vi "CreateDAQDict.vi"(8 "error in (no error)":errorcluster, 10 "IO Tasks[]":T1[](array[typedef])=[{"IO Type"=enum."DI", "TaskID"="DI_TaskID_C1", "IONames"=["DI1_00_Main Photohelic Pressure Low", "DI1_01_Main Photohelic Pressure High", "DI1_02_Main E-Stop Circuit OK", "DI1_03_EMO Circuit OK", "DI1_04_Nitrogen Top Valve Open", "DI1_05_Nitrogen Bottom Valve Open", "DI1_06_Nitrogen Pressure OK", "DI1_07_CDA Pressure OK", "DI1_08_Vacuum OK", "DI1_09_Aligner Home", "DI1_10_Aligner Reticle Present", "DI1_11_Main Door Interlock Solenoid Closed", "DI1_12_Main Door Closed", "DI1_13_Main Robot $ALARM_STOP", "DI1_14_Main Robot $IN_HOME", "DI1_15_Main Robot $PERI_RDY", "DI1_16_Main Robot $TCP_OPEN", "DI1_17_Main End Eff Open", "DI1_18_Main End Eff Closed", "DI1_19_Main Reticle Presence sensor-Arm-Right", "DI1_20_Spare_1", "DI1_21_Main Reticle Presence sensor-Arm-Left", "DI1_22_EXP1 XFR Reticle Present", "DI1_23_EXP2 XFR Reticle Present", "DI1_24_Main Robot $EXT (External Mode ON)", "DI1_25_Main Robot $PRO_ACT (Program Active)", "DI1_26_Main Robot $PRO_MOVE (Motion Active)", "DI1_27_Main Robot Spare1", "DI1_28_Main Robot Spare2", "DI1_29_Main Robot Spare3", "DI1_30_Spare_2", "DI1_31_Spare_3", "DI2_00_ASML_RSP LP 1 Pod Presence", "DI2_01_Spare_4", "DI2_02_ASML_RSP LP 2 Pod Presence", "DI2_03_Spare_5", "DI2_04_ASML_RSP LP 3 Pod Presence", "DI2_05_Spare_6", "DI2_06_Spare_7", "DI2_07_Manual Loadport 1 Pod Present", "DI2_08_Manual Loadport 1 Pod Capture", "DI2_09_Manual Loadport 1 Arm in Open Position", "DI2_10_Manual Loadport 1 Arm in Closed Position", "DI2_11_Manual Loadport 1 Lid Capture", "DI2_12_Manual Loadport 1 Door Closed", "DI2_13_Manual Loadport 1 Reticle Present", "DI2_14_Manual Loadport 1 Lid Present on Arm", "DI2_15_MLP Spare Input", "DI2_16_Pod Buffer Inbound Pod Present", "DI2_17_Pod Buffer Outbound Pod Present", "DI2_18_Pod Buffer Door Closed", "DI2_19_Pod Buffer Light Curtain OK", "DI2_20_Pod Buffer Light Curtain Misc Input", "DI2_21_Pod Buffer Gripper Pod Present", "DI2_22_Pod Buffer Gripper open", "DI2_23_Pod Buffer Gripper closed", "DI2_24_FFU Pressure sensor 1", "DI2_25_FFU Pressure sensor 2", "DI2_26_FFU Pressure sensor 3", "DI2_27_FFU Pressure sensor 4", "DI2_28_FFU Pressure sensor 5", "DI2_29_FFU Pressure sensor 6", "DI2_30_FFU Pressure sensor 7", "DI2_31_FFU Pressure sensor 8"], "ChPath"=["C1M1_9425_DI1/Port0/Line0", "C1M1_9425_DI1/Port0/Line1", "C1M1_9425_DI1/Port0/Line2", "C1M1_9425_DI1/Port0/Line3", "C1M1_9425_DI1/Port0/Line4", "C1M1_9425_DI1/Port0/Line5", "C1M1_9425_DI1/Port0/Line6", "C1M1_9425_DI1/Port0/Line7", "C1M1_9425_DI1/Port0/Line8", "C1M1_9425_DI1/Port0/Line9", "C1M1_9425_DI1/Port0/Line10", "C1M1_9425_DI1/Port0/Line11", "C1M1_9425_DI1/Port0/Line12", "C1M1_9425_DI1/Port0/Line13", "C1M1_9425_DI1/Port0/Line14", "C1M1_9425_DI1/Port0/Line15", "C1M1_9425_DI1/Port0/Line16", "C1M1_9425_DI1/Port0/Line17", "C1M1_9425_DI1/Port0/Line18", "C1M1_9425_DI1/Port0/Line19", "C1M1_9425_DI1/Port0/Line20", "C1M1_9425_DI1/Port0/Line21", "C1M1_9425_DI1/Port0/Line22", "C1M1_9425_DI1/Port0/Line23", "C1M1_9425_DI1/Port0/Line24", "C1M1_9425_DI1/Port0/Line25", "C1M1_9425_DI1/Port0/Line26", "C1M1_9425_DI1/Port0/Line27", "C1M1_9425_DI1/Port0/Line28", "C1M1_9425_DI1/Port0/Line29", "C1M1_9425_DI1/Port0/Line30", "C1M1_9425_DI1/Port0/Line31", "C1M2_9425_DI2/Port0/Line0", "C1M2_9425_DI2/Port0/Line1", "C1M2_9425_DI2/Port0/Line2", "C1M2_9425_DI2/Port0/Line3", "C1M2_9425_DI2/Port0/Line4", "C1M2_9425_DI2/Port0/Line5", "C1M2_9425_DI2/Port0/Line6", "C1M2_9425_DI2/Port0/Line7", "C1M2_9425_DI2/Port0/Line8", "C1M2_9425_DI2/Port0/Line9", "C1M2_9425_DI2/Port0/Line10", "C1M2_9425_DI2/Port0/Line11", "C1M2_9425_DI2/Port0/Line12", "C1M2_9425_DI2/Port0/Line13", "C1M2_9425_DI2/Port0/Line14", "C1M2_9425_DI2/Port0/Line15", "C1M2_9425_DI2/Port0/Line16", "C1M2_9425_DI2/Port0/Line17", "C1M2_9425_DI2/Port0/Line18", "C1M2_9425_DI2/Port0/Line19", "C1M2_9425_DI2/Port0/Line20", "C1M2_9425_DI2/Port0/Line21", "C1M2_9425_DI2/Port0/Line22", "C1M2_9425_DI2/Port0/Line23", "C1M2_9425_DI2/Port0/Line24", "C1M2_9425_DI2/Port0/Line25", "C1M2_9425_DI2/Port0/Line26", "C1M2_9425_DI2/Port0/Line27", "C1M2_9425_DI2/Port0/Line28", "C1M2_9425_DI2/Port0/Line29", "C1M2_9425_DI2/Port0/Line30", "C1M2_9425_DI2/Port0/Line31"], "Task Ref"=""}, {"IO Type"=enum."DI", "TaskID"="DI_TaskID_C2A", "IONames"=["DI3_00_Exp1 Photohelic Pressure Low", "DI3_01_Main Photohelic Pressure High", "DI3_02_Main E-Stop Circuit OK", "DI3_03_Spare_1", "DI3_04_Exp1 Door Interlock Solenoid Closed", "DI3_05_Exp1 Door Closed", "DI3_06_Spare_2", "DI3_07_Spare_3", "DI3_08_Spare_4", "DI3_09_Spare_5", "DI3_10_Exp1 End Eff Open", "DI3_11_Exp1 End Eff Closed", "DI3_12_Exp1 Reticle Presence sensor-Arm-Right", "DI3_13_Exp1 Robot $ALARM_STOP", "DI3_14_Exp1 Robot $IN_HOME", "DI3_15_Exp1 Robot $PERI_RDY", "DI3_16_Exp1 Robot $TCP_OPEN", "DI3_17_Exp1 Reticle Presence sensor-Arm-Left", "DI3_18_Exp1 FFU Pressure sensor 1", "DI3_19_Exp1 FFU Pressure sensor 2", "DI3_20_Exp1 FFU Pressure sensor 3", "DI3_21_Exp1 FFU Pressure sensor 4", "DI3_22_Exp1 FFU Pressure sensor 5", "DI3_23_Exp1 FFU Pressure sensor 6", "DI3_24_Exp1 Robot $EXT (External Mode ON)", "DI3_25_Exp1 Robot $PRO_ACT (Program Active)", "DI3_26_Exp1 Robot $PRO_MOVE (Motion Active)", "DI3_27_Exp1 FFU Pressure sensor 7", "DI3_28_Exp1 FFU Pressure sensor 8", "DI3_29_Exp1 output Spare 1", "DI3_30_Exp1 output Spare 2", "DI3_31_Exp1 output Spare 3"], "ChPath"=["C2AM1_9425_DI3/Port0/Line0", "C2AM1_9425_DI3/Port0/Line1", "C2AM1_9425_DI3/Port0/Line2", "C2AM1_9425_DI3/Port0/Line3", "C2AM1_9425_DI3/Port0/Line4", "C2AM1_9425_DI3/Port0/Line5", "C2AM1_9425_DI3/Port0/Line6", "C2AM1_9425_DI3/Port0/Line7", "C2AM1_9425_DI3/Port0/Line8", "C2AM1_9425_DI3/Port0/Line9", "C2AM1_9425_DI3/Port0/Line10", "C2AM1_9425_DI3/Port0/Line11", "C2AM1_9425_DI3/Port0/Line12", "C2AM1_9425_DI3/Port0/Line13", "C2AM1_9425_DI3/Port0/Line14", "C2AM1_9425_DI3/Port0/Line15", "C2AM1_9425_DI3/Port0/Line16", "C2AM1_9425_DI3/Port0/Line17", "C2AM1_9425_DI3/Port0/Line18", "C2AM1_9425_DI3/Port0/Line19", "C2AM1_9425_DI3/Port0/Line20", "C2AM1_9425_DI3/Port0/Line21", "C2AM1_9425_DI3/Port0/Line22", "C2AM1_9425_DI3/Port0/Line23", "C2AM1_9425_DI3/Port0/Line24", "C2AM1_9425_DI3/Port0/Line25", "C2AM1_9425_DI3/Port0/Line26", "C2AM1_9425_DI3/Port0/Line27", "C2AM1_9425_DI3/Port0/Line28", "C2AM1_9425_DI3/Port0/Line29", "C2AM1_9425_DI3/Port0/Line30", "C2AM1_9425_DI3/Port0/Line31"], "Task Ref"=""}, {"IO Type"=enum."DO", "TaskID"="DO_TaskID_C1", "IONames"=["DO1_00_Vacuum Circuit Enable", "DO1_01_Nitrogen Flow Valve Open", "DO1_02_Nitrogen Top Blow Off", "DO1_03_Nitrogen Bottom Blow Off", "DO1_04_Nitrogen Blow Off Exhaust Fan ON", "DO1_05_Signal Red Light", "DO1_06_Signal Amber Light", "DO1_07_Signal Green Light", "DO1_08_Signal Blue Light", "DO1_09_Robot Input spare 1", "DO1_10_Signal Flashing", "DO1_11_Door Interlock Solenoid Close", "DO1_12_Main Robot $CONF_MESS (Clear Error-Alarm)", "DO1_13_Main Robot $DRIVES_ON", "DO1_14_Main Robot $MOVE_ENABLE", "DO1_15_Main Robot $EXT_START (Start-Resume Program)", "DO1_16_Main Robot $DRIVES_OFF", "DO1_17_Robot Input Spare 2", "DO1_18_Robot Input Spare 3", "DO1_19_Robot Input Spare 4", "DO1_20_Robot Input Spare 5", "DO1_21_Pod Buffer Horiz Enable", "DO1_22_Pod Buffer Vert Enable", "DO1_23_Barcode Reader Backlight ON", "DO1_24_Digital Camera Image Capture", "DO1_25_BLIS ON", "DO1_26_Spare_1", "DO1_27_Spare_2", "DO1_28_Spare_3", "DO1_29_Spare_4", "DO1_30_Spare_5", "DO1_31_Spare_6", "DO2_00_Spare_7", "DO2_01_Spare_8", "DO2_02_Spare_9", "DO2_03_MLP1 Door Lock", "DO2_04_MLP1 Pod Capture", "DO2_05_MLP1 Lid Capture", "DO2_06_MLP1 Arm to Open position", "DO2_07_MLP1 Arm to Close position", "DO2_08_MLP1 Power On Indicator", "DO2_09_MLP1 Error Indicator", "DO2_10_MLP1 In Process Indicator", "DO2_11_Spare_10", "DO2_12_Spare_11", "DO2_13_Spare_12", "DO2_14_Spare_13", "DO2_15_Spare_14", "DO2_16_Spare_15", "DO2_17_Spare", "DO2_18_Spare", "DO2_19_Spare", "DO2_20_Spare", "DO2_21_Spare", "DO2_22_Spare", "DO2_23_Spare", "DO2_24_Spare", "DO2_25_Spare", "DO2_26_Spare", "DO2_27_Spare", "DO2_28_Spare", "DO2_29_Spare", "DO2_30_Spare", "DO2_31_Spare"], "ChPath"=["C1M3_9476_DO1/Port0/Line0", "C1M3_9476_DO1/Port0/Line1", "C1M3_9476_DO1/Port0/Line2", "C1M3_9476_DO1/Port0/Line3", "C1M3_9476_DO1/Port0/Line4", "C1M3_9476_DO1/Port0/Line5", "C1M3_9476_DO1/Port0/Line6", "C1M3_9476_DO1/Port0/Line7", "C1M3_9476_DO1/Port0/Line8", "C1M3_9476_DO1/Port0/Line9", "C1M3_9476_DO1/Port0/Line10", "C1M3_9476_DO1/Port0/Line11", "C1M3_9476_DO1/Port0/Line12", "C1M3_9476_DO1/Port0/Line13", "C1M3_9476_DO1/Port0/Line14", "C1M3_9476_DO1/Port0/Line15", "C1M3_9476_DO1/Port0/Line16", "C1M3_9476_DO1/Port0/Line17", "C1M3_9476_DO1/Port0/Line18", "C1M3_9476_DO1/Port0/Line19", "C1M3_9476_DO1/Port0/Line20", "C1M3_9476_DO1/Port0/Line21", "C1M3_9476_DO1/Port0/Line22", "C1M3_9476_DO1/Port0/Line23", "C1M3_9476_DO1/Port0/Line24", "C1M3_9476_DO1/Port0/Line25", "C1M3_9476_DO1/Port0/Line26", "C1M3_9476_DO1/Port0/Line27", "C1M3_9476_DO1/Port0/Line28", "C1M3_9476_DO1/Port0/Line29", "C1M3_9476_DO1/Port0/Line30", "C1M3_9476_DO1/Port0/Line31", "C1M4_9476_DO2/Port0/Line0", "C1M4_9476_DO2/Port0/Line1", "C1M4_9476_DO2/Port0/Line2", "C1M4_9476_DO2/Port0/Line3", "C1M4_9476_DO2/Port0/Line4", "C1M4_9476_DO2/Port0/Line5", "C1M4_9476_DO2/Port0/Line6", "C1M4_9476_DO2/Port0/Line7", "C1M4_9476_DO2/Port0/Line8", "C1M4_9476_DO2/Port0/Line9", "C1M4_9476_DO2/Port0/Line10", "C1M4_9476_DO2/Port0/Line11", "C1M4_9476_DO2/Port0/Line12", "C1M4_9476_DO2/Port0/Line13", "C1M4_9476_DO2/Port0/Line14", "C1M4_9476_DO2/Port0/Line15", "C1M4_9476_DO2/Port0/Line16", "C1M4_9476_DO2/Port0/Line17", "C1M4_9476_DO2/Port0/Line18", "C1M4_9476_DO2/Port0/Line19", "C1M4_9476_DO2/Port0/Line20", "C1M4_9476_DO2/Port0/Line21", "C1M4_9476_DO2/Port0/Line22", "C1M4_9476_DO2/Port0/Line23", "C1M4_9476_DO2/Port0/Line24", "C1M4_9476_DO2/Port0/Line25", "C1M4_9476_DO2/Port0/Line26", "C1M4_9476_DO2/Port0/Line27", "C1M4_9476_DO2/Port0/Line28", "C1M4_9476_DO2/Port0/Line29", "C1M4_9476_DO2/Port0/Line30", "C1M4_9476_DO2/Port0/Line31"], "Task Ref"=""}, {"IO Type"=enum."DO", "TaskID"="DO_TaskID_C2B", "IONames"=["DO3_00_Exp1 Door Lock Solenoid Close", "DO3_01_Spare", "DO3_02_Spare", "DO3_03_Spare", "DO3_04_Spare", "DO3_05_Spare", "DO3_06_Exp1 Input Spare 1", "DO3_07_Exp1 Input Spare 2", "DO3_08_Exp1 Input Spare 3", "DO3_09_Exp1 Input Spare 4", "DO3_10_Exp1 Input Spare 5", "DO3_11_Spare", "DO3_12_Exp1 Robot $CONF_MESS (Clear Error-Alarm)", "DO3_13_Exp1 Robot $DRIVES_ON", "DO3_14_Exp1 Robot $MOVE_ENABLE", "DO3_15_Exp1 Robot $EXT_START (Start-Resume Program)", "DO3_16_Exp1 Robot $DRIVES_OFF", "DO3_17_Spare", "DO3_18_Spare", "DO3_19_Spare", "DO3_20_Spare", "DO3_21_Spare", "DO3_22_Spare", "DO3_23_Spare", "DO3_24_Spare", "DO3_25_Spare", "DO3_26_Spare", "DO3_27_Spare", "DO3_28_Spare", "DO3_29_Spare", "DO3_30_Spare", "DO3_31_Spare"], "ChPath"=["C2BM1_9476_DO3/Port0/Line0", "C2BM1_9476_DO3/Port0/Line1", "C2BM1_9476_DO3/Port0/Line2", "C2BM1_9476_DO3/Port0/Line3", "C2BM1_9476_DO3/Port0/Line4", "C2BM1_9476_DO3/Port0/Line5", "C2BM1_9476_DO3/Port0/Line6", "C2BM1_9476_DO3/Port0/Line7", "C2BM1_9476_DO3/Port0/Line8", "C2BM1_9476_DO3/Port0/Line9", "C2BM1_9476_DO3/Port0/Line10", "C2BM1_9476_DO3/Port0/Line11", "C2BM1_9476_DO3/Port0/Line12", "C2BM1_9476_DO3/Port0/Line13", "C2BM1_9476_DO3/Port0/Line14", "C2BM1_9476_DO3/Port0/Line15", "C2BM1_9476_DO3/Port0/Line16", "C2BM1_9476_DO3/Port0/Line17", "C2BM1_9476_DO3/Port0/Line18", "C2BM1_9476_DO3/Port0/Line19", "C2BM1_9476_DO3/Port0/Line20", "C2BM1_9476_DO3/Port0/Line21", "C2BM1_9476_DO3/Port0/Line22", "C2BM1_9476_DO3/Port0/Line23", "C2BM1_9476_DO3/Port0/Line24", "C2BM1_9476_DO3/Port0/Line25", "C2BM1_9476_DO3/Port0/Line26", "C2BM1_9476_DO3/Port0/Line27", "C2BM1_9476_DO3/Port0/Line28", "C2BM1_9476_DO3/Port0/Line29", "C2BM1_9476_DO3/Port0/Line30", "C2BM1_9476_DO3/Port0/Line31"], "Task Ref"=""}]) -> (0 "error out":errorcluster, 2 "IO Tasks[] out":T1[](array[typedef]), 3 "DAQ IO Dict":T2, 5 "TaskIDs":string[](array[string]))   [LabVIEW 2020, in "DAQDict.lvlib"]
doc: "Developed by Kevin Thompson\nkevin@thompsonengineering.net\n\nCopyright 2021\nThompson Engineering, LLC"
uses:
  DAQDict.lvlib
  support/IONameNode--cluster.ctl
  support/IO Task--cluster.ctl
  support/IO Task Dict Node--cluster.ctl
  <vilib>/DAQmx/write.llb/DAQmx Write (Digital 1D Bool NChan 1Samp 1Line).vi
  <vilib>/DAQmx/read.llb/DAQmx Read (Digital 1D Bool NChan 1Samp 1Line).vi
  <vilib>/TELLC/Dynamic CVT API/TD Dynamic CVT DVR--ref.ctl
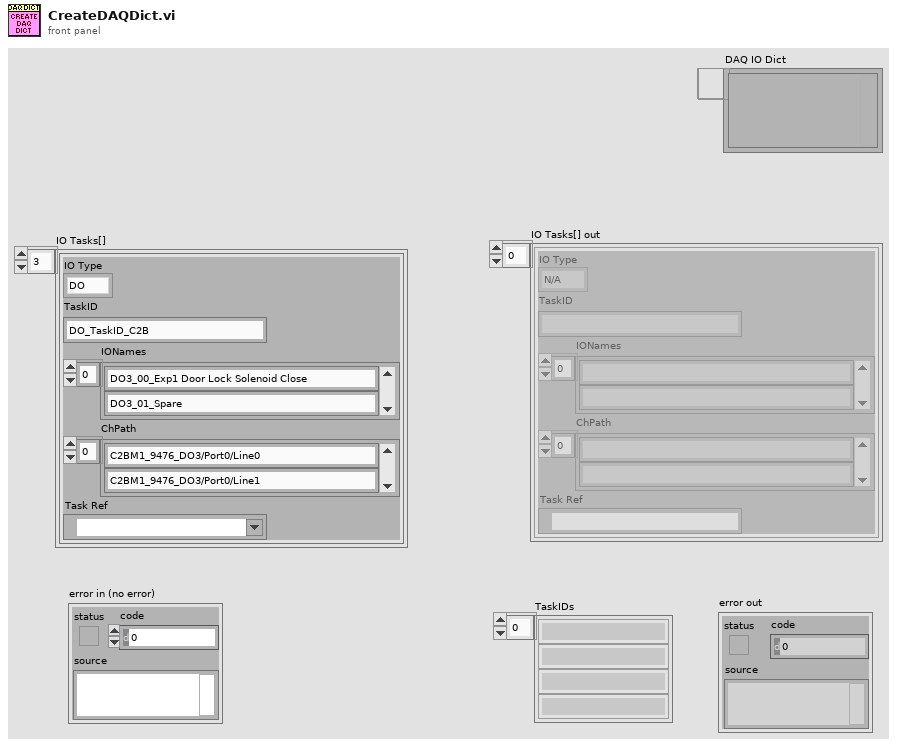
[diagram p1: front panel]
types:
  T1 = typedef "IO Task--cluster.ctl" = cluster{"IO Type":enum16{"N/A", "DI", "DO"}, "TaskID":string, "IONames":string[], "ChPath":string[], "Task Ref":refnum<k21>}
  T2 = typedef "TD Dynamic CVT DVR--ref.ctl" = refnum<data-value>
  T3 = typedef "IO Task Dict Node--cluster.ctl" = cluster{"IO Type":enum16{"N/A", "DI", "DO"}, "IONames":string[], "values":bool[], "IO Task":T1}
  T4 = typedef "IONameNode--cluster.ctl" = cluster{"IOName":string, "value":bool, "IO Type":enum16{"N/A", "DI", "DO"}, "TaskID":string, "data Idx":i32}
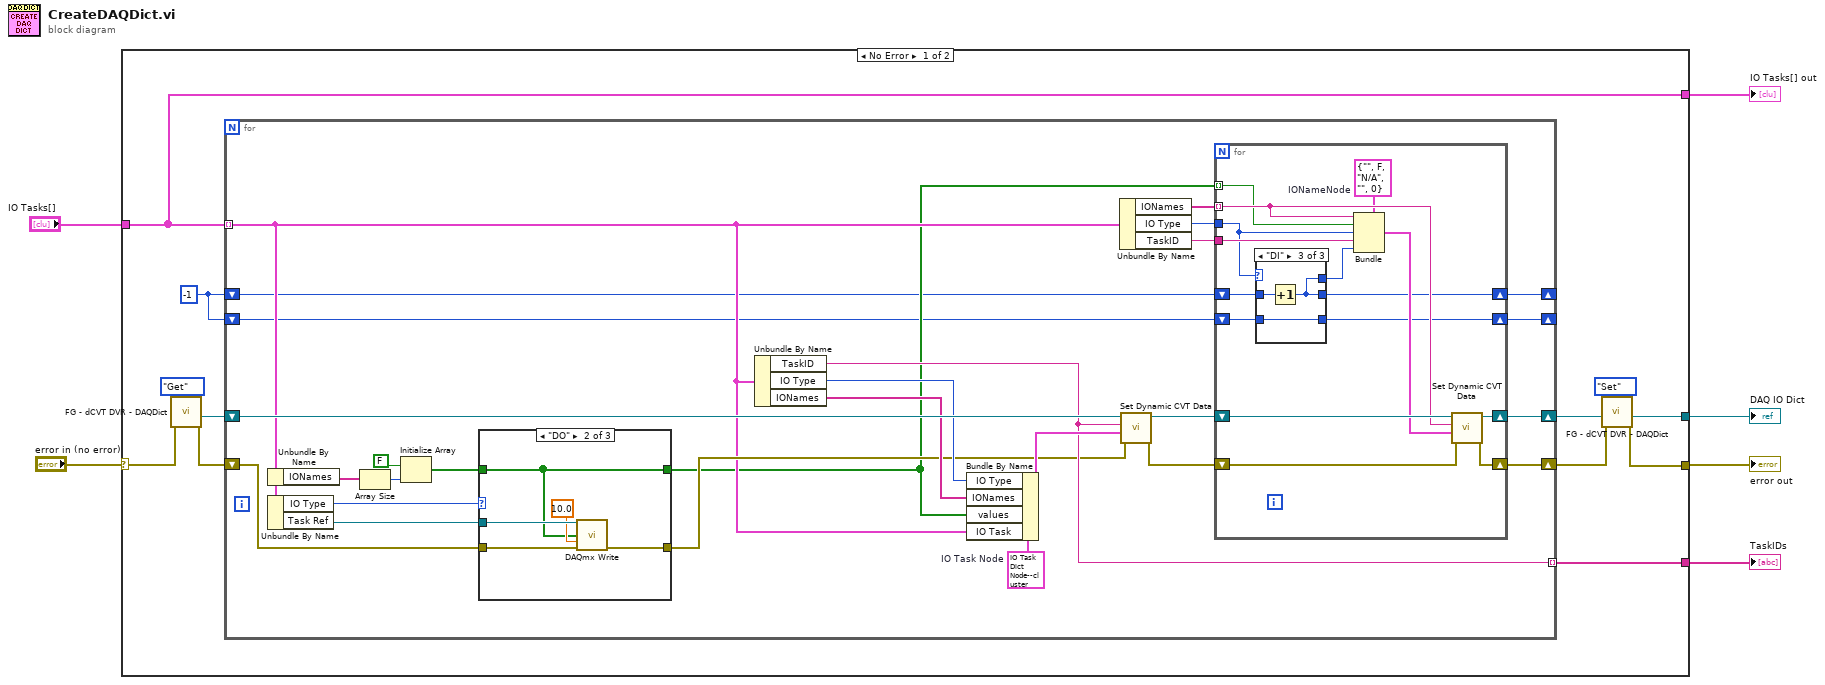
[diagram p0: block diagram]
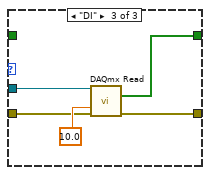
[diagram p3: hidden frame]
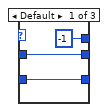
[diagram p4: hidden frame]
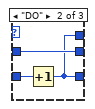
[diagram p5: hidden frame]
diagram:
  n1 = case shown="No Error" "error in (no error)" {
    selector: "error in (no error)" -> [w10 w82]
    tunnel: [w16 _] -> w6
    tunnel: [w14 w82] -> w5
    tunnel: "IO Tasks[]" -> [w9 w81]
    tunnel: [w9 w81] -> w2
    tunnel: [w8 _] -> w1
    frame No Error {
      w7 = -1
      n2 = call "FG - dCVT DVR - DAQDict.vi"("error in (no error)"=w10, "Action (Get)"=enum16{"Init", "Get", "Set"}."Get") -> ("dCVT DAQDict out"=w12:T2, "error out"=w11:errorcluster)  [unwired: 7 in]
      n3 = for {
        shift-right: [w42] -> w15
        shift-left: w11 -> [w32]
        shift-right: [w41] -> w18
        shift-left: w12 -> [w45]
        tunnel: w9 -> [w24] mode=indexing
        tunnel: [w33] -> w8 mode=indexing
        shift-right: [w21] -> _
        shift-left: w7 -> [w22]
        shift-right: [w19] -> _
        shift-left: w7 -> [w20]
        w37 = T3 {"IO Type"=enum."N/A", "IONames"=[], "values"=[], "IO Task"={"IO Type"=enum."N/A", "TaskID"="", "IONames"=[], "ChPath"=[], "Task Ref"=""}}  # IO Task Node
        n4 = Unbundle By Name(w24) -> ("IONames"=w27:string[])
        n5 = Unbundle By Name(w24) -> ("IO Type"=w26:enum16{"N/A", "DI", "DO"}, "Task Ref"=w30:refnum<k21>)
        n6 = Array Size(array=w27) -> (size(s)=w29:i32)
        n7 = Initialize Array(FALSE, w29) -> (w25:bool[])
        n8 = case shown="\"DO\"" w26 {
          tunnel: w32 -> [w46 w51 w54]
          tunnel: [w46 w50 w53] -> w31
          tunnel: w30 -> [_ w49 w55]
          tunnel: w25 -> [_ w47 _]
          tunnel: [_ w47 w52] -> w23
          frame "N/A", Default {
          }
          frame "DO" {
            n9 = call-poly <vilib>:"DAQmx Write.vi"("task/channels in"=w49, "data"=w47, "timeout"=10.0, "error in"=w51) -> ("error out"=w50:errorcluster)  [unwired: 9 in, 2 out]
          }
          frame "DI" {
            n10 = call-poly <vilib>:"DAQmx Read.vi"("task/channels in"=w55, "timeout"=10.0, "error in"=w54) -> ("data"=w52:bool[], "error out"=w53:errorcluster)  [unwired: 10 in, 1 out]
          }
        }
        n11 = Unbundle By Name(w24) -> ("TaskID"=w33:string, "IO Type"=w35:enum16{"N/A", "DI", "DO"}, "IONames"=w36:string[])
        n12 = Bundle By Name(cluster=w37, "IO Type"=w35, "IONames"=w36, "values"=w23, "IO Task"=w24) -> (w34:T3)
        n13 = Unbundle By Name(w24) -> ("IONames"=w40:string[], "IO Type"=w39:enum16{"N/A", "DI", "DO"}, "TaskID"=w38:string)
        n14 = call <vilib>:"Set Dynamic CVT Data.vi"("error in (no error)"=w31, "value"=w34, "DataName"=w33, "dCVT DVR"=w45) -> ("error out"=w43:errorcluster, "dCVT DVR out"=w44:T2)  [unwired: 5 in, 1 out]
        n15 = for {
          shift-right: [w68] -> w41
          shift-left: w44 -> [w71]
          shift-right: [w69] -> w42
          shift-left: w43 -> [w70]
          tunnel: w40 -> [w66] mode=indexing
          tunnel: w39 -> [w62]
          tunnel: w38 -> [w67]
          tunnel: w23 -> [w63] mode=indexing
          shift-right: [w59] -> w21
          shift-left: w22 -> [w61]
          shift-right: [w58] -> w19
          shift-left: w20 -> [w60]
          w65 = T4 {"IOName"="", "value"=FALSE, "IO Type"=enum."N/A", "TaskID"="", "data Idx"=0}  # IONameNode
          n16 = case shown="\"DI\"" w62 {
            tunnel: w61 -> [w74 w76 w80]
            tunnel: w60 -> [w73 w77 w79]
            tunnel: [w74 w76 w78] -> w59
            tunnel: [w73 w75 w79] -> w58
            tunnel: [-1 w75 w78] -> w57
            frame Default {
            }
            frame "DO" {
              n17 = Increment(x=w77) -> (x+1=w75:i32)
            }
            frame "DI" {
              n18 = Increment(x=w80) -> (x+1=w78:i32)
            }
          }
          n19 = Bundle(cluster=w65, "IOName"=w66, "value"=w63, "IO Type"=w62, "TaskID"=w67, "data Idx"=w57) -> (w64:T4)
          n20 = call <vilib>:"Set Dynamic CVT Data.vi"("error in (no error)"=w70, "value"=w64, "DataName"=w66, "dCVT DVR"=w71) -> ("error out"=w69:errorcluster, "dCVT DVR out"=w68:T2)  [unwired: 5 in, 1 out]
        }
      }
      n21 = call "FG - dCVT DVR - DAQDict.vi"("dCVT DAQDict"=w18, "error in (no error)"=w15, "Action (Get)"=enum16{"Init", "Get", "Set"}."Set") -> ("dCVT DAQDict out"=w16:T2, "error out"=w14:errorcluster)  [unwired: 6 in]
    }
    frame Error {
    }
  }
  "DAQ IO Dict" <- w6
  "error out" <- w5
  "IO Tasks[] out" <- w2
  "TaskIDs" <- w1
